vi "Temperature Monitor.vi"() -> ()   [LabVIEW 2012]
doc: "该VI是LabVIEW核心课程1中练习的答案。\n\n该VI使用While循环和移位寄存器进行均值计算。无需硬件。"
panel:
  in  "停止按钮":bool
  out "温度历史":dbl(graph)
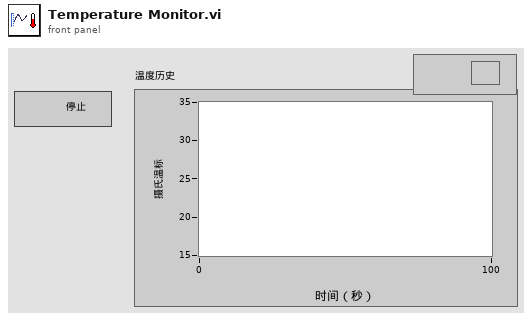
[diagram p1: front panel]
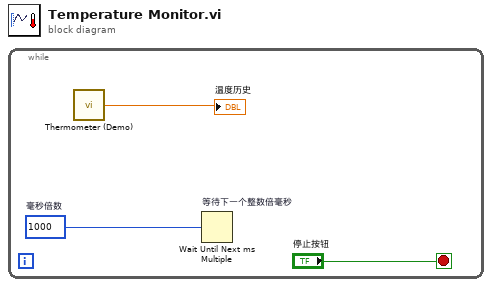
[diagram p0: block diagram]
diagram:
  n1 = while {
    stop <- "停止按钮" stop-if-true
    w3 = u32 1000  # 毫秒倍数
    n2 = call "Thermometer (Demo).vi"() -> ("温度值"=→"温度历史":dbl)  [unwired: 1 in]
    n3 = Wait Until Next ms Multiple "等待下一个整数倍毫秒"(millisecond multiple=w3) -> ()  [unwired: 1 out]
  }
